vi "Format VCOM to System Definition Path.vi"(8 "error in (no error)":errorcluster, 11 "VCOM Signal":string) -> (0 "error out":errorcluster, 3 "System Definition Path":string)   [LabVIEW 2025]
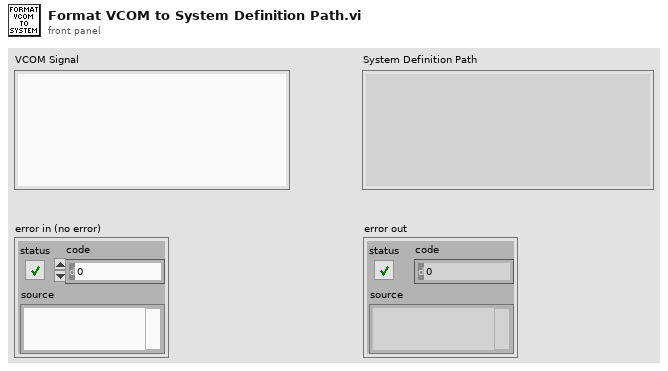
[diagram p1: front panel]
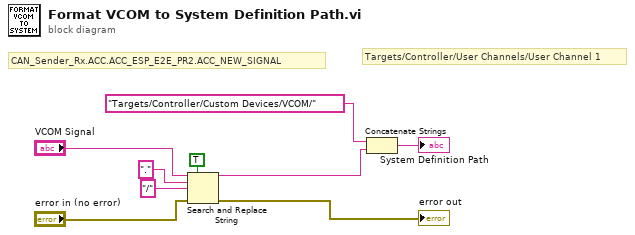
[diagram p0: block diagram]
diagram:
  # "CAN_Sender_Rx.ACC.ACC_ESP_E2E_PR2.ACC_NEW_SIGNAL"
  # "Targets/Controller/User Channels/User Channel 1"
  n1 = Search and Replace String(replace all?=TRUE ("replace all? (F)"), input string="VCOM Signal", search string=".", replace string="/" ("search string"), error in="error in (no error)") -> (result string=w4:string, error out=→"error out":errorcluster)  [unwired: 3 in, 2 out]
  n2 = Concatenate Strings("Targets/Controller/Custom Devices/VCOM/" ("string"), w4) -> (→"System Definition Path":string)
